vi "SetSN.vi"(8 "error in (no error)":errorcluster, 9 "DUT":u32, 10 "SN":string, 11 "reference in":refnum<class "TestView_Tree_Single.lvclass">) -> (0 "error out":errorcluster, 3 "reference in":refnum<class "TestView_Tree_Single.lvclass">)   [LabVIEW 2022 SP3, in "TestView_Tree_Single.lvlib" / "TestView_Tree_Single.lvclass"]
uses:
  TestView_Tree_Single.lvclass
  Components/TestView_Base.lvlibp/ViewStatus.ctl
  Components/TestView_Base.lvlibp/TestView_Base.lvclass
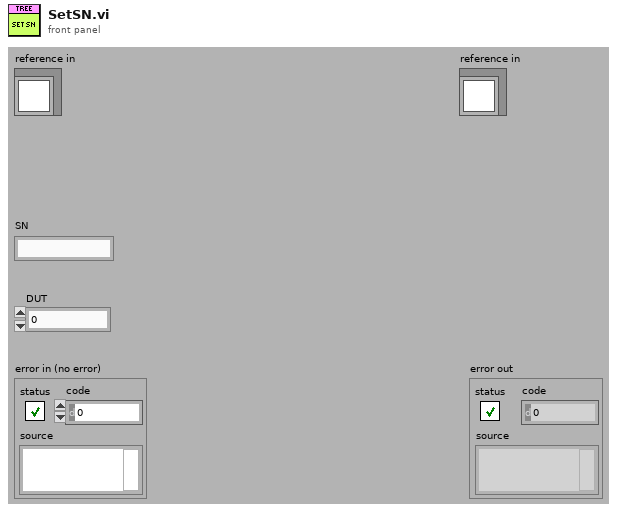
[diagram p1: front panel]
types:
  T1 = typedef "TestView_Base.lvlibp/TestView_Base.lvclass/ViewStatus.ctl" = enum16{"Testing", "Ready", "Logout", "Login", "PASS", "FAIL", "FAULT", "ABORTED"}
  T2 = typedef "TestView_Tree_Single.lvlib/TestView_Tree_Single.lvclass/ObjectAttributes.ctl" = cluster{"Front Panel":refnum<vi>, "Last_Item":string, "Config":T3, "Title":string, "User":string, "TreeRef":refnum<vi>, "Active DUT":i32, "Status":T1, "SN":string, "Spec":string}
  T3 = typedef "TestView_Tree_Single.lvlib/TestView_Tree_Single.lvclass/Config.ctl" = cluster{"default":string}
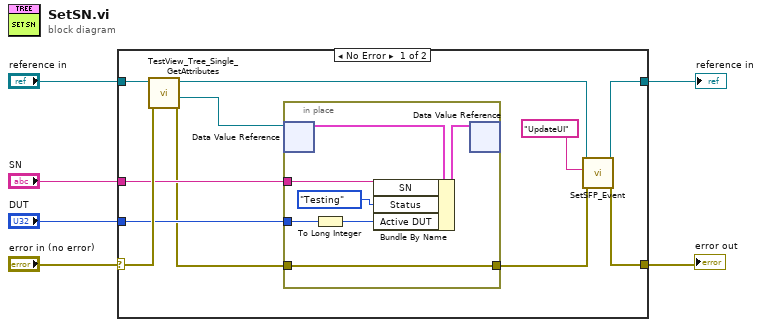
[diagram p0: block diagram]
diagram:
  n1 = case shown="No Error" "error in (no error)" {
    selector: "error in (no error)" -> [w17 w26]
    tunnel: [w7 w26] -> w5
    tunnel: [w13 w25] -> w3
    tunnel: "reference in" -> [w16 w25]
    tunnel: "SN" -> [w11 _]
    tunnel: "DUT" -> [w10 _]
    frame No Error {
      n2 = call "TestView_Tree_Single_GetAttributes.vi"("error in (no error)"=w17, "reference in"=w16) -> ("error out"=w9:errorcluster, "DataRef"=w12:refnum<data-value>, "reference out"=w14:refnum<class "TestView_Tree_Single.lvclass">)  [unwired: 6 in, 1 out]
      n3 = in-place {
        in-place-border: w11 -> [w18]
        in-place-border: w10 -> [w22]
        in-place-border: [w21] -> w8
        in-place-border: w9 -> [w21]
        n4 = in-place-dvr #1(w12) -> (w23:T2)  [unwired: 1 out]
        n5 = To Long Integer(number=w22) -> (32bit integer=w20:i32)
        n6 = Bundle By Name(cluster=w23, "SN"=w18, "Status"=ViewStatus."Testing", "Active DUT"=w20) -> (w24:T2)
        n7 = in-place-dvr #1(w24) -> ()  [unwired: 2 out]
      }
      n8 = call-dynamic "SetSFP_Event.vi"("error in (no error)"=w8, "msg"="UpdateUI", "reference in"=w14) -> ("error out"=w7:errorcluster, "reference out"=w13:refnum<class "TestView_Tree_Single.lvclass">)  [unwired: 7 in]
    }
    frame Error {
    }
  }
  "error out" <- w5
  "reference in" <- w3
